vi "KTable Test Context Dependent Rings.vi"() -> ()   [LabVIEW 2015]
uses:
  KTable/KTable.xctl
panel:
  in  "Array":cluster{"Value1":string, "Value2":string}[](array[cluster])=[{"Value1"="Alpha1", "Value2"=""}]
  in  "stop":bool
  in  "KTable":u16(xcontrol)
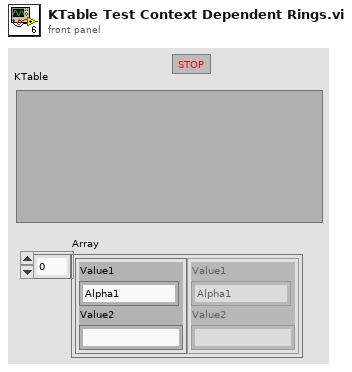
[diagram p1: front panel]
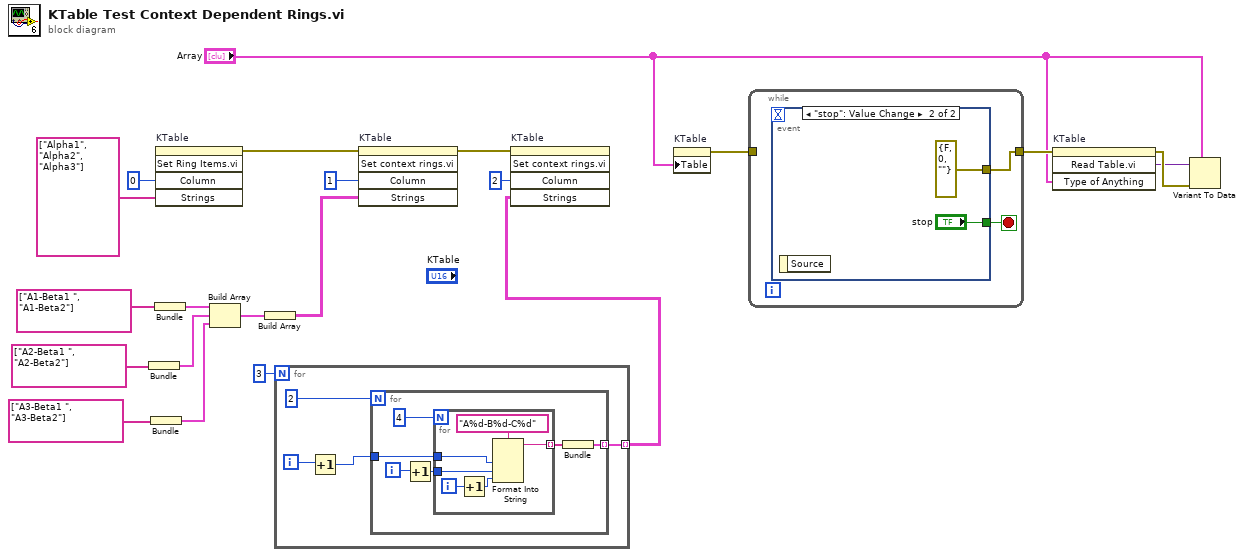
[diagram p0: block diagram]
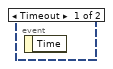
[diagram p2: hidden frame]
diagram:
  n1 = Bundle("Strings"=string[] ["A2-Beta1 ", "A2-Beta2"]) -> (w11:cluster{"Strings":string[]})  [unwired: 1 in]
  n2 = Bundle("Strings"=string[] ["A3-Beta1 ", "A3-Beta2"]) -> (w9:cluster{"Strings":string[]})  [unwired: 1 in]
  n3 = Bundle("Strings"=string[] ["A1-Beta1 ", "A1-Beta2"]) -> (w13:cluster{"Strings":string[]})  [unwired: 1 in]
  n4 = invoke on="KTable" class="KTable (strict)" method="Set Ring Items.vi"("Column"=0, "Strings"=string[] ["Alpha1", "Alpha2", "Alpha3"]) -> (error out=w8:errorcluster)  [unwired: 3 in, 4 out]
  n5 = Build Array(w13, w11, w9) -> (w6:cluster{"Strings":string[]}[])
  n6 = Build Array(w6) -> (w5:cluster{"Strings":string[]}[][])
  n7 = for {
    N: 3 -> [_]
    tunnel: [w22] -> w1 mode=indexing
    i -> [w24]
    n8 = Increment(x=w24) -> (x+1=w23:i32)
    n9 = for {
      N: 2 -> [_]
      tunnel: w23 -> [w28]
      tunnel: [w26] -> w22 mode=indexing
      i -> [w30]
      n10 = Increment(x=w30) -> (x+1=w29:i32)
      n11 = for {
        N: 4 -> [_]
        tunnel: w29 -> [w34]
        tunnel: w28 -> [w33]
        tunnel: [w32] -> w27 mode=indexing
        i -> [w36]
        n12 = Increment(x=w36) -> (x+1=w35:i32)
        n13 = Format Into String(format string="A%d-B%d-C%d", w33, w34, w35) -> (resulting string=w32:string)  [unwired: 2 in, 1 out]
      }
      n14 = Bundle(w27) -> (w26:cluster{string[]})  [unwired: 1 in]
    }
  }
  n15 = invoke on="KTable" class="KTable (strict)" method="Set context rings.vi"(error in=w8, "Column"=1, "Strings"=w5) -> (error out=w3:errorcluster)  [unwired: 2 in, 4 out]
  n16 = invoke on="KTable" class="KTable (strict)" method="Set context rings.vi"(error in=w3, "Column"=2, "Strings"=w1) -> ()  [unwired: 2 in, 5 out]
  n17 = property on="KTable" class="KTable (strict)"("Table"="Array") -> (error out=w15:errorcluster)  [unwired: 2 in, 1 out]
  n18 = while {
    tunnel: [w38] -> w21
    tunnel: w15 -> [_]
    stop <- w39 stop-if-true
    n19 = event shown="[1] \"stop\": Value Change" {
      selector: _ -> [_ _]
      dyn-events: _ -> [_ _]
      timeout: _ -> [_ _]
      tunnel: [_ "stop"] -> w39
      tunnel: [_ errorcluster {"status"=FALSE, "code"=0, "source"=""} ("error constant")] -> w38
      event Timeout {
        n20 = event-data() -> ()  [unwired: 1 in, 1 out]
      }
      event "stop": Value Change {
        n21 = event-data() -> ()  [unwired: 1 in, 1 out]
      }
    }
  }
  n22 = invoke on="KTable" class="KTable (strict)" method="Read Table.vi"(error in=w21, "Type of Anything"="Array") -> (error out=w20:errorcluster, "Read Table.vi"=w19:variant)  [unwired: 2 in, 2 out]
  n23 = Variant To Data(error in=w20, type="Array", Variant=w19) -> ()  [unwired: 2 out]
